vi "read_attributes.vi"(8 "error in (no error)":errorcluster, 11 "FeatureAgglomeration in":refnum<class "FeatureAgglomeration.lvclass">) -> (0 "error out":errorcluster, 2 "attributes":T1, 3 "FeatureAgglomeration out":refnum<class "FeatureAgglomeration.lvclass">)   [LabVIEW 2020, in "FeatureAgglomeration.lvclass"]
uses:
  FeatureAgglomeration.lvclass
  Controls/feature_agglomeration_attributes.ctl
  FeatureAgglomeration.lvclass/FeatureAgglomeration.ctl
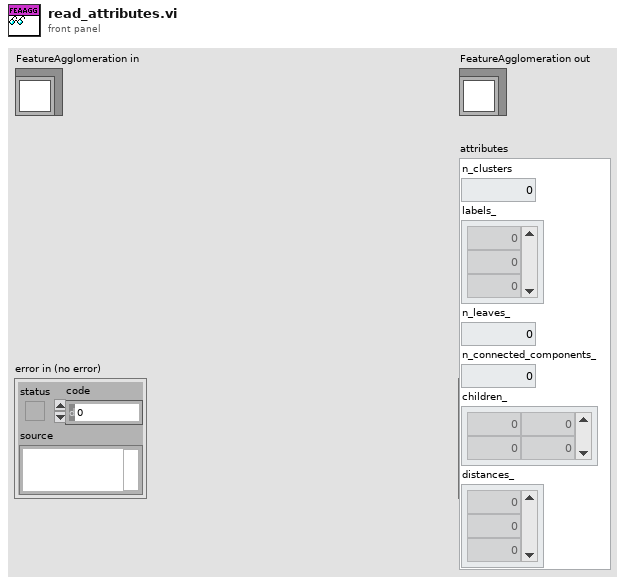
[diagram p1: front panel]
types:
  T1 = typedef "feature_agglomeration_attributes.ctl" = cluster{"n_clusters":dbl, "labels_":dbl[], "n_leaves_":dbl, "n_connected_components_":dbl, "children_":dbl[][], "distances_":dbl[]}
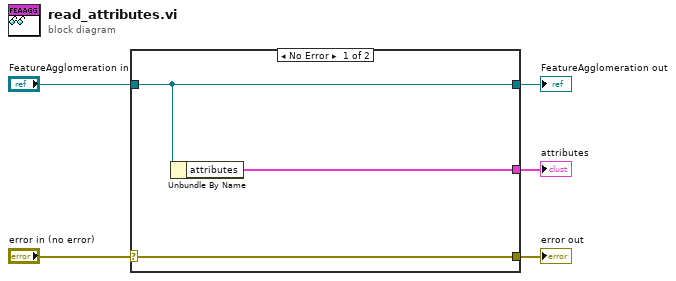
[diagram p0: block diagram]
diagram:
  n1 = case shown="No Error" "error in (no error)" {
    selector: "error in (no error)" -> [w8 w9]
    tunnel: [w8 w9] -> w4
    tunnel: [w7 w10] -> w2
    tunnel: "FeatureAgglomeration in" -> [w7 w10]
    tunnel: [w6 _] -> w1
    frame No Error {
      n2 = Unbundle By Name(w7) -> ("attributes"=w6:T1)
    }
    frame Error {
    }
  }
  "error out" <- w4
  "FeatureAgglomeration out" <- w2
  "attributes" <- w1
